vi "ResponseStreaming RouteGuide Test.vi"() -> ()   [LabVIEW 2019, in "route_guide_client.lvlib"]
uses:
  route_guide_client.lvlib
  RPC Messages/routeguide_Rectangle.ctl
  RPC Messages/routeguide_Point.ctl
  RPC Messages/routeguide_Feature.ctl
  <vilib>/gRPC/LabVIEW gRPC Library/grpc-lvsupport-release.lvlib
panel:
  out "error out":errorcluster
  out "Response Data":T1[](array[typedef])
  in  "Request Data":T3={"lo"={"latitude"=0, "longitude"=0}, "hi"={"latitude"=10, "longitude"=10}}
  in  "Server Address":string="localhost:50051"
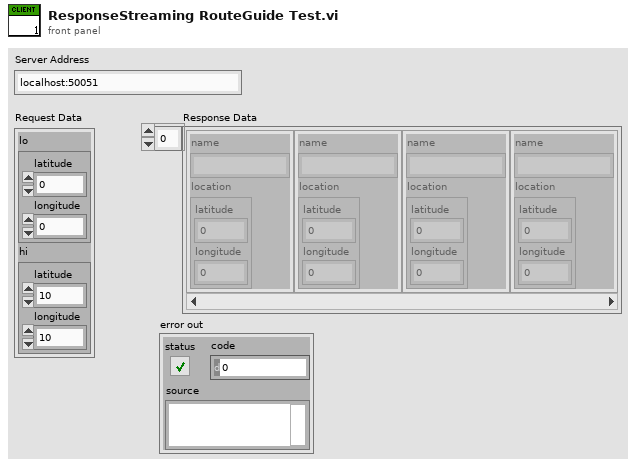
[diagram p1: front panel]
types:
  T1 = typedef "route_guide_client.lvlib/routeguide_Feature.ctl" = cluster{"name":string, "location":T2}
  T2 = typedef "route_guide_client.lvlib/routeguide_Point.ctl" = cluster{"latitude":i32, "longitude":i32}
  T3 = typedef "route_guide_client.lvlib/routeguide_Rectangle.ctl" = cluster{"lo":T2, "hi":T2}
  T4 = typedef "grpc-lvsupport-release.lvlib/grpcId.ctl" = u64
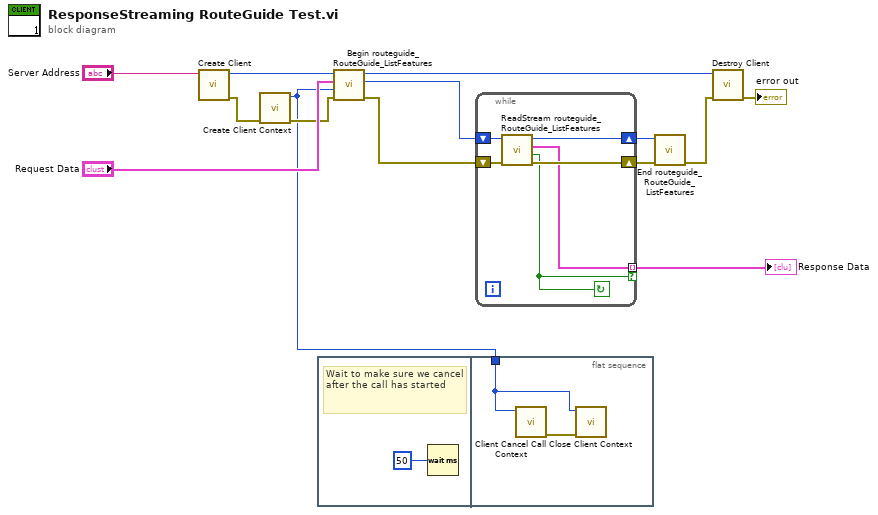
[diagram p0: block diagram]
diagram:
  n1 = call "Create Client.vi"("address"="Server Address") -> ("error out"=w3:errorcluster, "gRPC ID Out"=w13:T4)  [unwired: 9 in]
  n2 = call <vilib>:"Create Client Context.vi"("error in (no error)"=w3) -> ("error out"=w2:errorcluster, "ContextID out"=w1:T4)  [unwired: 9 in]
  n3 = flat-sequence {
    tunnel: w1 -> [w16]
    frame #0 {
      # "Wait to make sure we cancel after the call has started"
      n4 = Wait (ms)(milliseconds to wait=u32 50) -> ()  [unwired: 1 out]
    }
    frame #1 {
      n5 = call <vilib>:"Client Cancel Call Context.vi"("Call ID in"=w16) -> ("error out"=w17:errorcluster)  [unwired: 10 in]
      n6 = call <vilib>:"Close Client Context.vi"("error in (no error)"=w17, "ContextID"=w16) -> ()  [unwired: 9 in, 1 out]
    }
  }
  n7 = call "Begin routeguide_RouteGuide_ListFeatures.vi"("error in"=w2, "contextId"=w1, "Request Data"="Request Data", "gRPC ID"=w13) -> ("error out"=w11:errorcluster, "Call Id Out"=w10:T4, "gRPC ID out"=w7:T4)  [unwired: 5 in]
  n8 = while {
    shift-right: [w20] -> w8
    shift-left: w11 -> [w23]
    shift-right: [w21] -> w9
    shift-left: w10 -> [w22]
    tunnel: [w19] -> w5 mode=indexing if=w18
    stop <- w18 continue-if-true
    n9 = call "ReadStream routeguide_RouteGuide_ListFeatures.vi"("error in"=w23, "Call ID in"=w22) -> ("error out"=w20:errorcluster, "Success"=w18:bool, "Response Data"=w19:T1, "Call ID"=w21:T4)  [unwired: 6 in]
  }
  "Response Data" <- w5
  n10 = call "End routeguide_RouteGuide_ListFeatures.vi"("error in"=w8, "Call ID in"=w9) -> ("error out"=w6:errorcluster)  [unwired: 8 in, 1 out]
  n11 = call "Destroy Client.vi"("error in"=w6, "gRPC ID"=w7) -> ("error out"=→"error out":errorcluster)  [unwired: 9 in]
